vi "long_cmd_write.vi"(5 "COM":bool, 6 "dwLen":u32, 7 "VISA name":refnum<visa-resource-name>, 8 "error in":errorcluster, 9 "dwAddr2":u32, 10 "dwAddr1":u32, 11 "vd_cmd_long_header_t":T1) -> (0 "error out":errorcluster, 3 "return":i32)   [LabVIEW 2016]
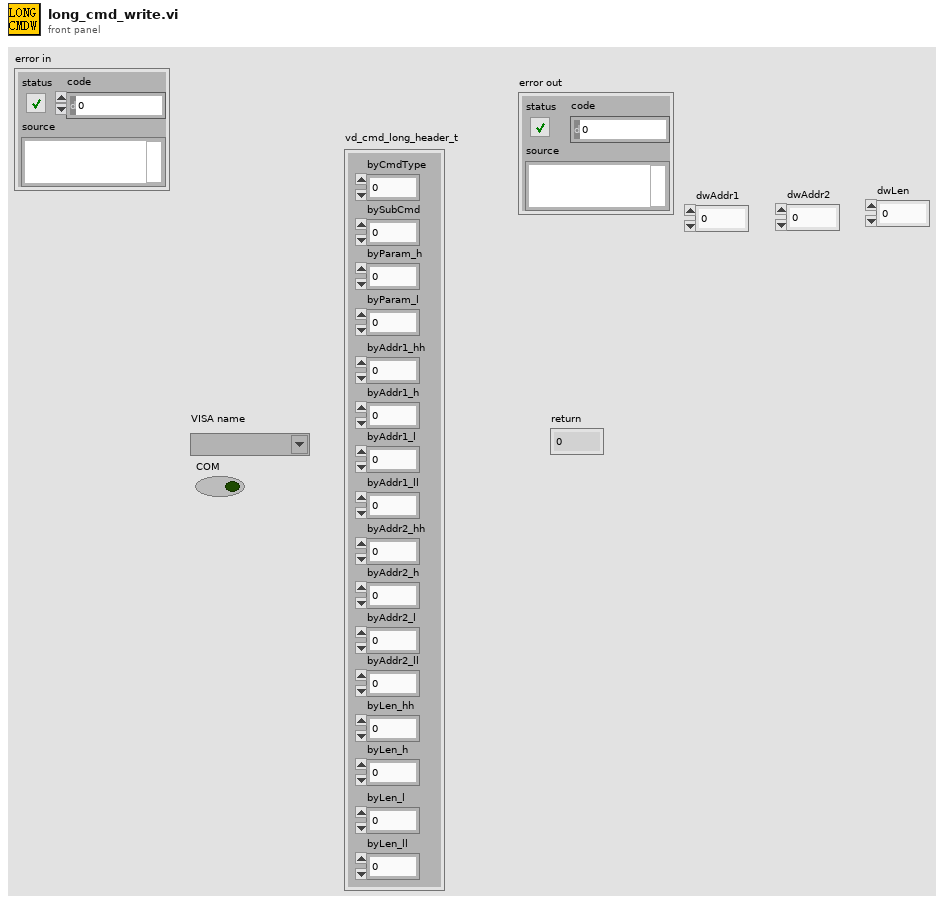
[diagram p1: front panel]
types:
  T1 = cluster{"byCmdType":u8, "bySubCmd":u8, "byParam_h":u8, "byParam_l":u8, "byAddr1_hh":u8, "byAddr1_h":u8, "byAddr1_l":u8, "byAddr1_ll":u8, "byAddr2_hh":u8, "byAddr2_h":u8, "byAddr2_l":u8, "byAddr2_ll":u8, "byLen_hh":u8, "byLen_h":u8, "byLen_l":u8, "byLen_ll":u8}
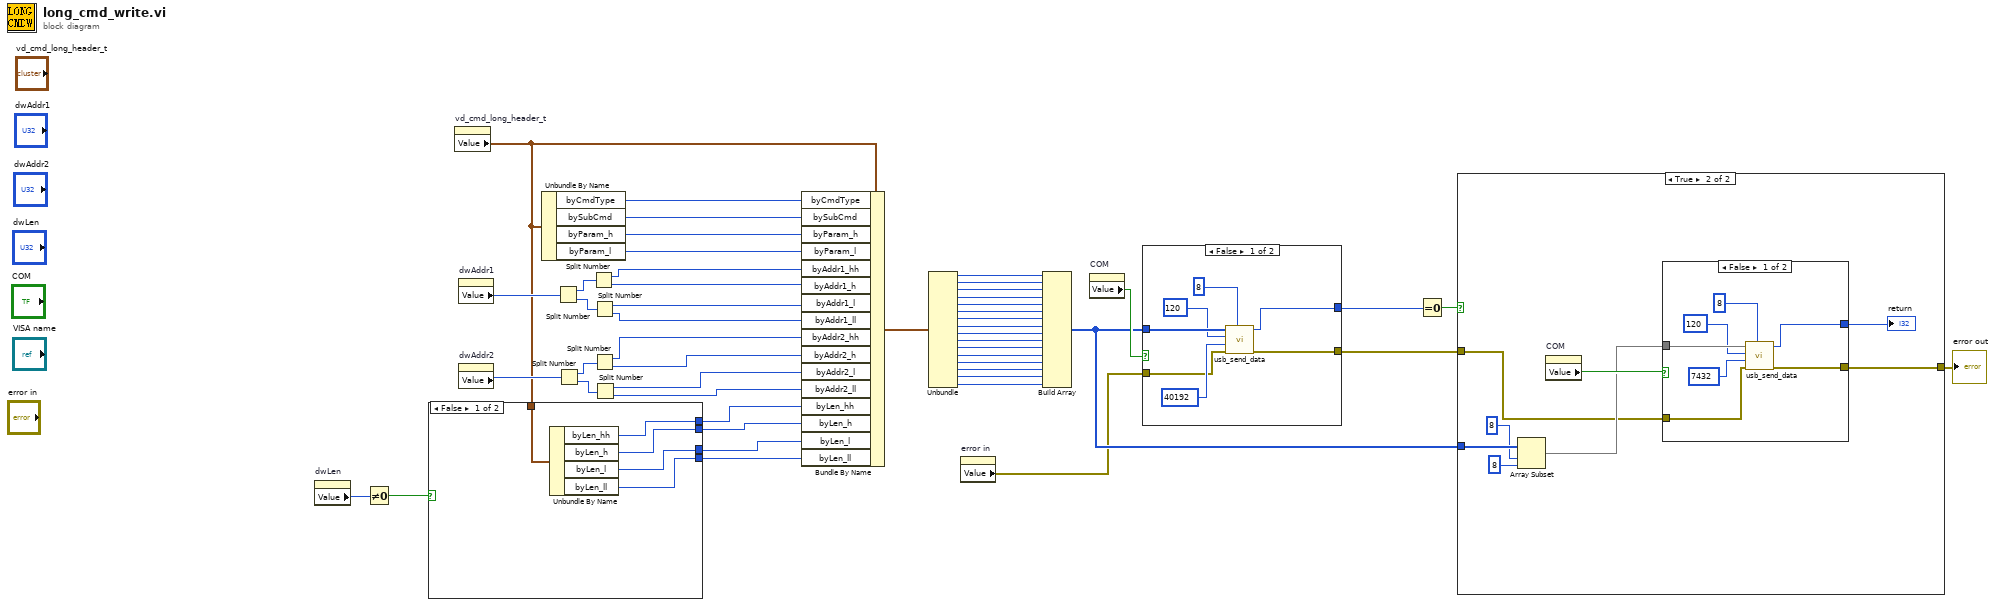
[diagram p0: block diagram]
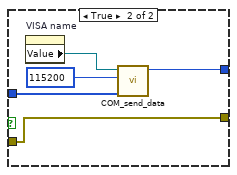
[diagram p2: hidden frame]
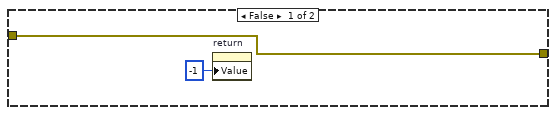
[diagram p3: hidden frame]
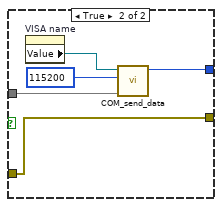
[diagram p4: hidden frame]
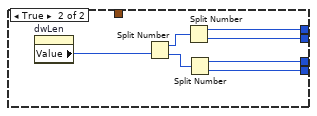
[diagram p5: hidden frame]
diagram:
  n1 = property on="dwLen" class="DigNum (strict)"() -> ("Value"=w49:u32)  [unwired: 2 in, 2 out]
  n2 = Not Equal To 0?(x=w49) -> (x != 0?=w26:bool)
  n3 = property on="vd_cmd_long_header_t" class="Clust (strict)"() -> ("Value"=w25:T1)  [unwired: 2 in, 2 out]
  n4 = case shown="False" w26 {
    tunnel: [w53 w58] -> w30
    tunnel: [w52 w57] -> w29
    tunnel: [w51 w56] -> w28
    tunnel: [w50 w55] -> w27
    tunnel: w25 -> [w54 _]
    frame False {
      n5 = Unbundle By Name(w54) -> ("byLen_hh"=w53:u8, "byLen_h"=w52:u8, "byLen_l"=w51:u8, "byLen_ll"=w50:u8)
    }
    frame True {
      n6 = property on="dwLen" class="DigNum (strict)"() -> ("Value"=w59:u32)  [unwired: 2 in, 2 out]
      n7 = Split Number(x=w59) -> (hi(x)=w61:u16, lo(x)=w60:u16)
      n8 = Split Number(x=w61) -> (hi(x)=w58:u8, lo(x)=w57:u8)
      n9 = Split Number(x=w60) -> (hi(x)=w56:u8, lo(x)=w55:u8)
    }
  }
  n10 = property on="dwAddr1" class="DigNum (strict)"() -> ("Value"=w46:u32)  [unwired: 2 in, 2 out]
  n11 = property on="dwAddr2" class="DigNum (strict)"() -> ("Value"=w43:u32)  [unwired: 2 in, 2 out]
  n12 = Unbundle By Name(w25) -> ("byCmdType"=w42:u8, "bySubCmd"=w41:u8, "byParam_h"=w40:u8, "byParam_l"=w39:u8)
  n13 = Split Number(x=w46) -> (hi(x)=w48:u16, lo(x)=w47:u16)
  n14 = Split Number(x=w43) -> (hi(x)=w44:u16, lo(x)=w45:u16)
  n15 = Split Number(x=w48) -> (hi(x)=w38:u8, lo(x)=w37:u8)
  n16 = Split Number(x=w47) -> (hi(x)=w36:u8, lo(x)=w35:u8)
  n17 = Split Number(x=w44) -> (hi(x)=w34:u8, lo(x)=w33:u8)
  n18 = Split Number(x=w45) -> (hi(x)=w32:u8, lo(x)=w31:u8)
  n19 = Bundle By Name(cluster=w25, "byCmdType"=w42, "bySubCmd"=w41, "byParam_h"=w40, "byParam_l"=w39, "byAddr1_hh"=w38, "byAddr1_h"=w37, "byAddr1_l"=w36, "byAddr1_ll"=w35, "byAddr2_hh"=w34, "byAddr2_h"=w33, "byAddr2_l"=w32, "byAddr2_ll"=w31, "byLen_hh"=w30, "byLen_h"=w29, "byLen_l"=w28, "byLen_ll"=w27) -> (w24:T1)
  n20 = Unbundle(w24) -> ("byCmdType"=w23:u8, "bySubCmd"=w22:u8, "byParam_h"=w21:u8, "byParam_l"=w20:u8, "byAddr1_hh"=w19:u8, "byAddr1_h"=w18:u8, "byAddr1_l"=w17:u8, "byAddr1_ll"=w16:u8, "byAddr2_hh"=w15:u8, "byAddr2_h"=w14:u8, "byAddr2_l"=w13:u8, "byAddr2_ll"=w12:u8, "byLen_hh"=w11:u8, "byLen_h"=w10:u8, "byLen_l"=w9:u8, "byLen_ll"=w8:u8)
  n21 = property on="error in" class="Clust (strict)"() -> ("Value"=w3:errorcluster)  [unwired: 2 in, 2 out]
  n22 = Build Array(w23, w22, w21, w20, w19, w18, w17, w16, w15, w14, w13, w12, w11, w10, w9, w8) -> (w4:u8[])
  n23 = property on="COM" class="Bool (strict)"() -> ("Value"=w7:bool)  [unwired: 2 in, 2 out]
  n24 = case shown="False" w7 {
    tunnel: w4 -> [w68 w73]
    tunnel: [w64 w70] -> w5
    tunnel: [w63 w69] -> w2
    tunnel: w3 -> [w62 w69]
    frame False {
      n25 = call "usb_send_data.vi"("byVdCmdHeaderLen"=u16 8, "error in"=w62, "I2C_VD_BUFFER_RW"=u16 40192, "I2C_SLAVE_ID"=u8 120, "data"=w68) -> ("error out"=w63:errorcluster, "return"=w64:i32)  [unwired: 5 in]
    }
    frame True {
      n26 = property on="VISA name" class="VISAName"() -> ("Value"=w71:refnum<visa-resource-name>)  [unwired: 2 in, 2 out]
      n27 = call "COM_send_data.vi"("data"=w73, "baud rate (9600)"=u32 115200, "VISA name"=w71) -> ("return"=w70:i32)  [unwired: 8 in]
    }
  }
  n28 = Equal To 0?(x=w5) -> (x = 0?=w6:bool)
  n29 = case shown="True" w6 {
    tunnel: w4 -> [_ w82]
    tunnel: w2 -> [w74 w77]
    tunnel: [w74 w76] -> w1
    frame False {
      n30 = property on="return" class="DigNum (strict)"("Value"=-1 ("return")) -> ()  [unwired: 2 in, 2 out]
    }
    frame True {
      n31 = Array Subset(array=w82, index=8, length=8) -> (w79:u8[])
      n32 = property on="COM" class="Bool (strict)"() -> ("Value"=w83:bool)  [unwired: 2 in, 2 out]
      n33 = case shown="False" w83 {
        tunnel: w79 -> [w90 w95]
        tunnel: [w86 w92] -> w78
        tunnel: w77 -> [w85 w91]
        tunnel: [w84 w91] -> w76
        frame False {
          n34 = call "usb_send_data.vi"("byVdCmdHeaderLen"=u16 8, "error in"=w85, "I2C_VD_BUFFER_RW"=u16 7432, "I2C_SLAVE_ID"=u8 120, "data"=w90) -> ("error out"=w84:errorcluster, "return"=w86:i32)  [unwired: 5 in]
        }
        frame True {
          n35 = property on="VISA name" class="VISAName"() -> ("Value"=w93:refnum<visa-resource-name>)  [unwired: 2 in, 2 out]
          n36 = call "COM_send_data.vi"("data"=w95, "baud rate (9600)"=u32 115200, "VISA name"=w93) -> ("return"=w92:i32)  [unwired: 8 in]
        }
      }
      "return" <- w78
    }
  }
  "error out" <- w1
